vi "FTW-Endpoint-Multipart-Read.vi"(0 "FTW Endpoint":refnum<class "FTW-Endpoint.lvclass">, 5 "Timeout":i32 format="%dmsec", 11 "error in":errorcluster) -> (4 "FTW Endpoint out":refnum<class "FTW-Endpoint.lvclass">, 6 "Message Received":T1, 8 "Timed out?":bool, 15 "error out":errorcluster)   [LabVIEW 2013, in "FTW-Endpoint.lvclass"]
uses:
  FTW-Endpoint.lvclass
  Payload/FTW-MessagePayload.ctl
  FTW-Endpoint.lvclass/FTW-Endpoint.ctl
panel:
  # "Inputs"
  # "Outputs"
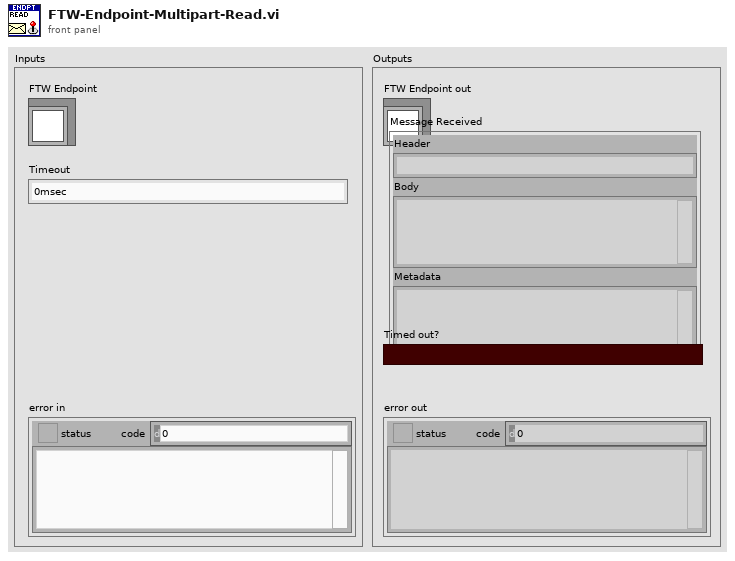
[diagram p1: front panel]
types:
  T1 = typedef "FTW-MessagePayload.ctl" = cluster{"Header":string, "Body":string, "Metadata":string}
  T2 = typedef "FTW-Message.ctl" = cluster{"Header":string, "Body":string, "Metadata":string}
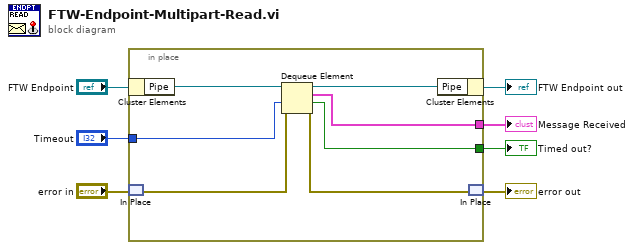
[diagram p0: block diagram]
diagram:
  n1 = in-place {
    in-place-border: "Timeout" -> [w13]
    in-place-border: [w11] -> w4
    in-place-border: [w10] -> w3
    n2 = in-place-cluster #1("FTW Endpoint") -> ("Pipe"=w14:refnum<queue>)
    n3 = in-place-match #2("error in") -> (w9:errorcluster)
    n4 = Dequeue Element(queue=w14, timeout in ms (-1)=w13, error in (no error)=w9) -> (queue out=w12:refnum<queue>, element=w11:T2, timed out?=w10:bool, error out=w8:errorcluster)
    n5 = in-place-cluster #1("Pipe"=w12) -> (→"FTW Endpoint out":refnum<class "FTW-Endpoint.lvclass">)
    n6 = in-place-match #2(w8) -> (→"error out":errorcluster)
  }
  "Message Received" <- w4
  "Timed out?" <- w3
